vi "ZLIB Move Raw File__ogtk.vi"(7 "zip Refnum":T1, 8 "error in (no error)":errorcluster, 9 "file info":T3 {"file timestamp" format="%<%H:%M:%S\n%d/%m/%Y>T"; "external fa" format="%.0x"; "internal fa" format="%.0x"; "crc" format="%.0x"}, 10 "name":string, 11 "unzip Refnum":T2) -> (0 "error out":errorcluster, 3 "unzip Refnum out":T2, 5 "zip Refnum out":T1)   [LabVIEW 2020]
doc: "Copies the currently selected file from an unzip archive into another zip archive without the need for decompressing an recompressing it. This allows to copy even password protected files between archives and in this way the new file in the zip archive will inherit the password from the original file."
uses:
  <userlib>/_OpenG.lib/lvzip/lvzip.llb/ZLIB Unzip Handle__ogtk.ctl
  <userlib>/_OpenG.lib/lvzip/lvzip.llb/ZLIB Zip Handle__ogtk.ctl
  <userlib>/_OpenG.lib/lvzip/lvzip.llb/ZLIB File Info__ogtk.ctl
panel:
  # "Please visit http://www.OpenG.org to learn about the\nOpen Source LabVIEW software movement.\n\nNOTICE -- YOU MUST LEAVE THIS NOTICE IN PLACE.  PER THE TERMS OF THE LICENSE BELOW, YOU MAY SUBLICENSE THIS SOFTWARE \nIN ANY WAY THAT DOES NOT CONFLICT WITH THIS LICENSE.\n\n### BSD License (http://www.opensource.org/licenses/bsd-license.php) Begin ###\n \nCopyright (C) 2008 Rolf Kalbermatter rolf.kalbermatter@citeng.com\n\nAll rights reserved.\n\nRedistribution and use in source and binary forms, with or without modification, are permitted provided that the following conditions are met:\n\n    * Redistributions of source code must retain the above copyright notice, this list of conditions and the following disclaimer.\n    * Redistributions in binary form must reproduce the above copyright notice, this list of conditions and the following disclaimer in the \n       documentation and/or other materials provided with the distribution.\n    * Neither the name of SciWare, James Kring, Inc., nor the names of its contributors may be used to endorse or promote products derived \n       from this software without specific prior written permission.\n\nTHIS SOFTWARE IS PROVIDED BY THE COPYRIGHT HOLDERS AND CONTRIBUTORS \"AS IS\" AND ANY EXPRESS OR IMPLIED WARRANTIES, \nINCLUDING, BUT NOT LIMITED TO, THE IMPLIED WARRANTIES OF MERCHANTABILITY AND FITNESS FOR A PARTICULAR PURPOSE ARE \nDISCLAIMED. IN NO EVENT SHALL THE COPYRIGHT OWNER OR CONTRIBUTORS BE LIABLE FOR ANY DIRECT, INDIRECT, INCIDENTAL,\n SPECIAL, EXEMPLARY, OR CONSEQUENTIAL DAMAGES (INCLUDING, BUT NOT LIMITED TO, PROCUREMENT OF SUBSTITUTE GOODS OR \nSERVICES; LOSS OF USE, DATA, OR PROFITS; OR BUSINESS INTERRUPTION) HOWEVER CAUSED AND ON ANY THEORY OF LIABILITY, \nWHETHER IN CONTRACT, STRICT LIABILITY, OR TORT (INCLUDING NEGLIGENCE OR OTHERWISE) ARISING IN ANY WAY OUT OF THE USE \nOF THIS SOFTWARE, EVEN IF ADVISED OF THE POSSIBILITY OF SUCH DAMAGE.\n\n### BSD License End ###"
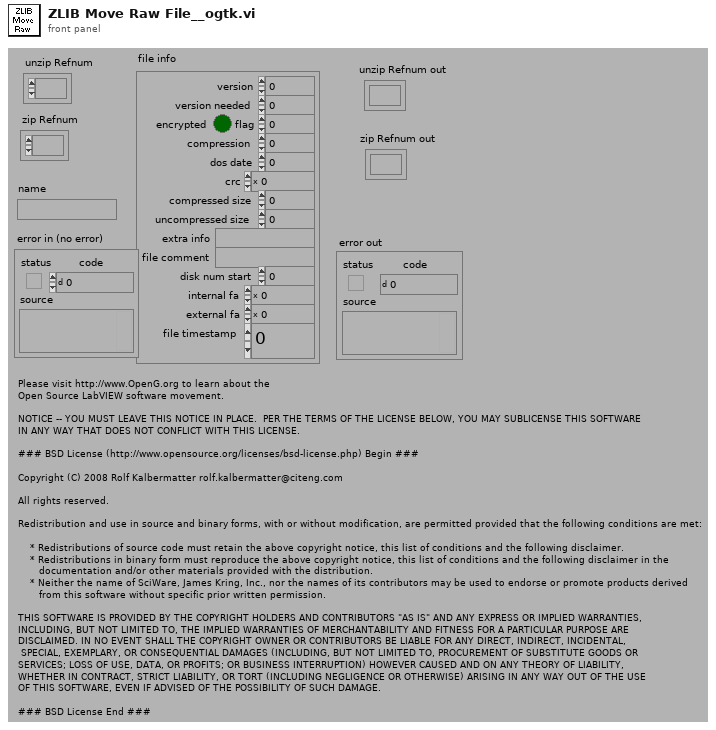
[diagram p1: front panel]
types:
  T1 = typedef "ZLIB Zip Handle__ogtk.ctl" = refnum<k1>
  T2 = typedef "ZLIB Unzip Handle__ogtk.ctl" = refnum<k1>
  T3 = typedef "ZLIB File Info__ogtk.ctl" = cluster{"version":u32, "version needed":u32, "encrypted":bool, "flag":u32, "compression":i32, "dos date":u32, "crc":u32, "compressed size":u32, "uncompressed size":u32, "extra info":string, "file comment":string, "disk num start":u32, "internal fa":u32, "external fa":u32, "file timestamp":u32}
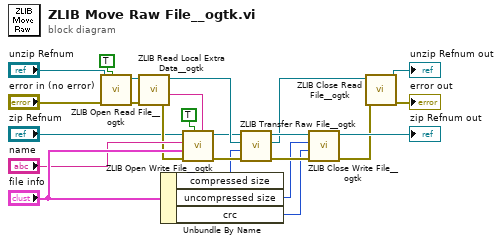
[diagram p0: block diagram]
diagram:
  n1 = call <userlib>:"ZLIB Open Read File__ogtk.vi"("raw mode (F)"=TRUE, "error in (no error)"="error in (no error)", "unzip Refnum"="unzip Refnum") -> ("error out"=w16:errorcluster, "unzip Refnum out"=w15:T2)  [unwired: 3 in, 2 out]
  n2 = call <userlib>:"ZLIB Read Local Extra Data__ogtk.vi"("error in (no error)"=w16, "unzip Refnum"=w15) -> ("error out"=w18:errorcluster, "local extra data"=w20:string, "unzip Refnum out"=w17:T2)  [unwired: 3 in]
  n3 = Unbundle By Name("file info") -> ("compressed size"=w3:u32, "uncompressed size"=w2:u32, "crc"=w1:u32)
  n4 = call <userlib>:"ZLIB Open Write File__ogtk.vi"("local extra data"=w20, "raw mode (F)"=TRUE, "error in (no error)"=w18, "file info"="file info", "filename"="name", "zip Refnum"="zip Refnum") -> ("error out"=w8:errorcluster, "zip Refnum out"=w9:T1)  [unwired: 4 in]
  n5 = call <userlib>:"ZLIB Transfer Raw File__ogtk.vi"("error in (no error)"=w8, "compressed size"=w3, "unzip Refnum"=w17, "zip Refnum"=w9) -> ("error out"=w7:errorcluster, "unzip Refnum out"=w5:T2, "zip Refnum out"=w11:T1)  [unwired: 2 in]
  n6 = call <userlib>:"ZLIB Close Write File__ogtk.vi"("error in (no error)"=w7, "crc32"=w1, "uncompressed size"=w2, "zip Refnum"=w11) -> ("error out"=w4:errorcluster, "zip Refnum out"=→"zip Refnum out":T1)  [unwired: 2 in]
  n7 = call <userlib>:"ZLIB Close Read File__ogtk.vi"("error in (no error)"=w4, "unzip Refnum"=w5) -> ("error out"=→"error out":errorcluster, "unzip Refnum out"=→"unzip Refnum out":T2)  [unwired: 8 in]
